vi "LDA_Probe.vi"(11 "LDA":refnum<class "LDA.lvclass">) -> (2 "Value String":string, 3 "Pause VI":bool)   [LabVIEW 2020, in "OpenLvVision_OpenCv.lvlib" / "LDA.lvclass"]
uses:
  LDA.lvclass
  _LvHelpers/EdvrObject/EdvrObject.lvclass
  C:/Users/lukas/Downloads/OpenLvVision_OpenCv/SourceCode/LabView/OpenLvVision_OpenCv/_LvHelpers/EdvrObject/EdvrObject.lvclass
  C:/Users/lukas/Downloads/OpenLvVision_OpenCv/SourceCode/LabView/OpenLvVision_OpenCv/CoreFunctionality/LDA/LDA/LDA.lvclass
panel:
  in  "Tab Control":enum32{"EigenValues", "EigenVectors"}(tab)
  out "EigenValues":dbl[](array[numeric])
  out "EigenVectors":dbl[][](array[numeric])
  out "Reference":u64 format="%.0x"
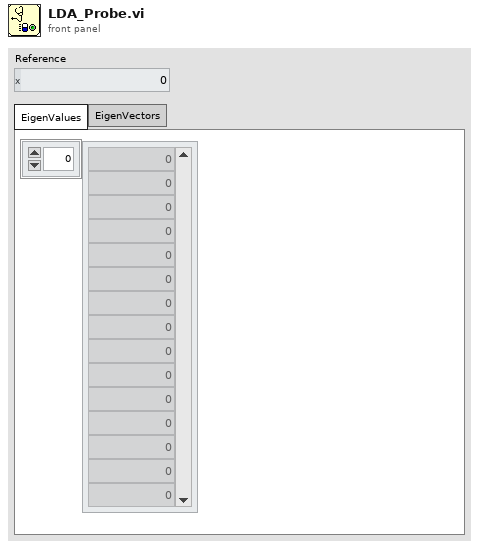
[diagram p1: front panel]
types:
  T1 = typedef "OpenLvVision_OpenCv.lvlib/EdvrObject.lvclass/Edvr.ctl" = refnum<data-value>
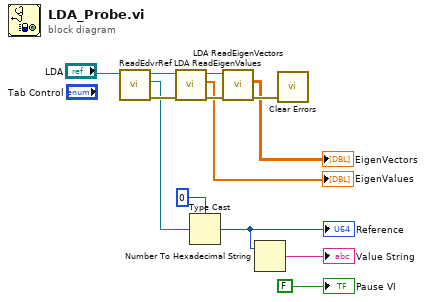
[diagram p0: block diagram]
diagram:
  n1 = call "ReadEdvrRef.vi"("EdvrObject in"="LDA") -> ("error out"=w5:errorcluster, "Edvr"=w1:T1, "EdvrObject out"=w6:refnum<class "LDA.lvclass">)  [unwired: 8 in]
  n2 = call "LDA ReadEigenValues.vi"("error in"=w5, "LDA"=w6) -> ("error out"=w3:errorcluster, "EigenValues"=→"EigenValues":dbl[], "LDA"=w4:refnum<class "LDA.lvclass">)  [unwired: 7 in]
  n3 = Type Cast(type=u64 0, x=w1) -> (*(type *) &x=w11:u64)
  "Reference" <- w11
  n4 = call "LDA ReadEigenVectors.vi"("error in"=w3, "LDA"=w4) -> ("error out"=w8:errorcluster, "EigenVectors"=→"EigenVectors":dbl[][])  [unwired: 7 in, 1 out]
  n5 = Number To Hexadecimal String(2:w11) -> (0:→"Value String":string)  [unwired: 1 in]
  n6 = call <vilib>:"Clear Errors.vi"("error in (no error)"=w8) -> ()  [unwired: 5 in, 2 out]
  "Pause VI" <- FALSE
